vi "Write Frequency.vi"(7 "PWM":refnum<class "PWM.lvclass">, 8 "error in (no error)":errorcluster, 10 "Frequency Hz":sgl, 11 "Session In":refnum<class "Session.lvclass">) -> (0 "error out":errorcluster, 3 "Session Out":refnum<class "Session.lvclass">)   [LabVIEW 2020, in "CTI.lvlib" / "PWM.lvclass"]
uses:
  PWM.lvclass
  PWM.lvclass/PWM.ctl
  GPIO/GPIO.lvclass
  Session/Session.lvclass
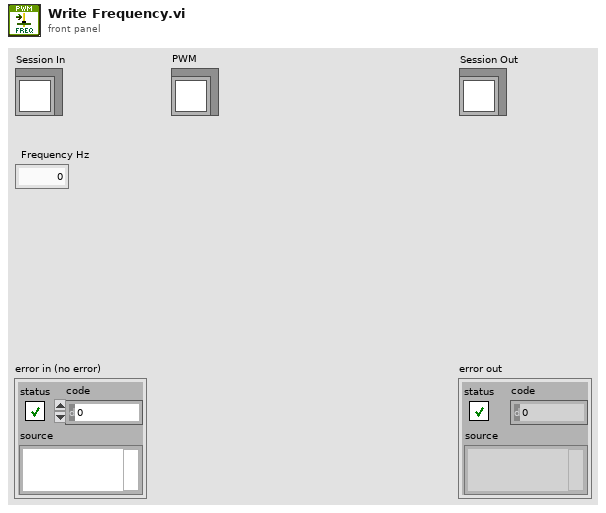
[diagram p1: front panel]
types:
  T1 = typedef "CTI.lvlib/GPIO Number.ctl" = i8
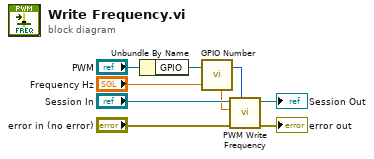
[diagram p0: block diagram]
diagram:
  n1 = Unbundle By Name("PWM") -> ("GPIO"=w3:refnum<class "GPIO.lvclass">)
  n2 = call "GPIO Number.vi"("GPIO in"=w3) -> ("GPIO #"=w2:T1)  [unwired: 6 in]
  n3 = call "PWM Write Frequency.vi"("GPIO #"=w2, "error in (no error)"="error in (no error)", "Frequency Hz"="Frequency Hz", "Session in"="Session In") -> ("error out"=→"error out":errorcluster, "Session out"=→"Session Out":refnum<class "Session.lvclass">)  [unwired: 6 in]
